vi "Show Hide Plot Legend.vi"(7 "show":bool, 8 "error in (no error)":errorcluster, 10 "view reference":refnum<vi>, 11 "graph reference":refnum<vi>) -> (0 "error out":errorcluster)   [LabVIEW 2021, in "UI Helpers.lvlib"]
uses:
  UI Helpers.lvlib
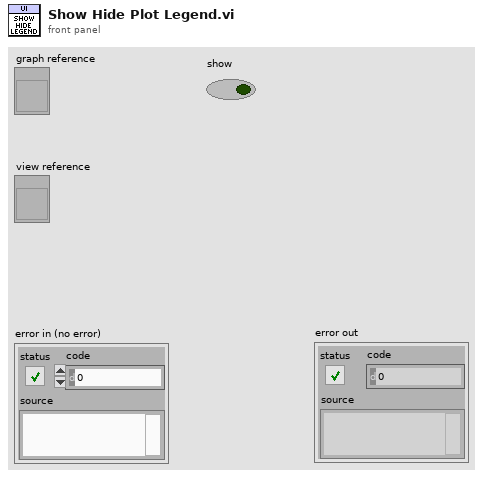
[diagram p1: front panel]
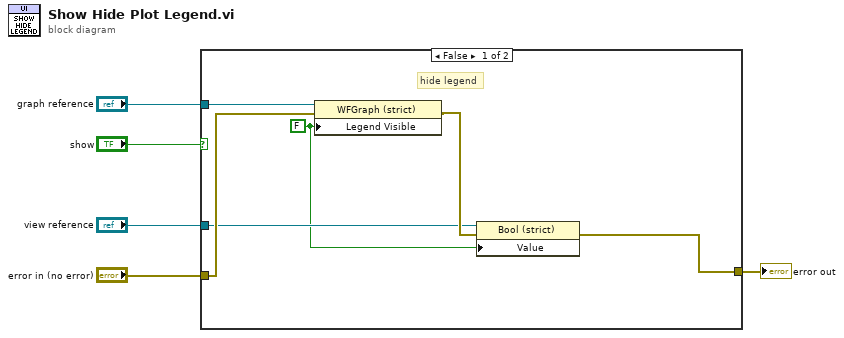
[diagram p0: block diagram]
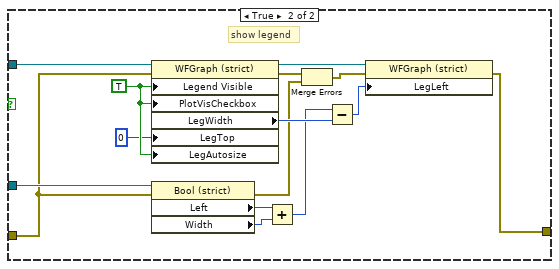
[diagram p2: hidden frame]
diagram:
  n1 = case shown="False" "show" {
    tunnel: "graph reference" -> [w11 w26]
    tunnel: "view reference" -> [w7 w18]
    tunnel: "error in (no error)" -> [w10 w16]
    tunnel: [w8 w12] -> w1
    frame False {
      w6 = FALSE ("Legend:Visible")
      # "hide legend"
      n2 = property on="Property Node" class="WFGraph (strict)"(reference=w11, error in=w10, "Legend Visible"=w6) -> (error out=w9:errorcluster)  [unwired: 1 out]
      n3 = property class="Bool (strict)"(reference=w7, error in=w9, "Value"=w6) -> (error out=w8:errorcluster)  [unwired: 1 out]
    }
    frame True {
      w25 = TRUE ("Legend:Visible")
      # "show legend"
      n4 = property on="Property Node" class="WFGraph (strict)"(reference=w26, error in=w16, "Legend Visible"=w25, "PlotVisCheckbox"=w25, "LegTop"=0 ("Legend:Position:Top"), "LegAutosize"=w25) -> (reference out=w23:refnum<vi>, error out=w15:errorcluster, "LegWidth"=w22:u32)
      n5 = property on="Property Node" class="Bool (strict)"(reference=w18, error in=w16) -> (error out=w14:errorcluster, "Left"=w20:i32, "Width"=w19:u32)  [unwired: 1 out]
      n6 = Add(x=w20, y=w19) -> (x+y=w17:u32)
      n7 = Merge Errors(w15, w14) -> (w13:errorcluster)
      n8 = Subtract(x=w17, y=w22) -> (x-y=w21:u32)
      n9 = property on="Property Node" class="WFGraph (strict)"(reference=w23, error in=w13, "LegLeft"=w21) -> (error out=w12:errorcluster)  [unwired: 1 out]
    }
  }
  "error out" <- w1
